vi "Receive Head Tail Location (SubVI).vi"() -> (3 "HT Location":u64[](array[numeric]))   [LabVIEW 2015]
uses:
  <vilib>/rvi/interface/RandomDataEmulation/niFpgaRandomDataHandleErrors.vi
  <vilib>/rvi/DataTransferAndStorage/Container/XNode/niFpgaContainer.xnode
  <vilib>/rvi/interface/RandomDataEmulation/nirviRandomDataFpgaReadWriteTemplate.vi
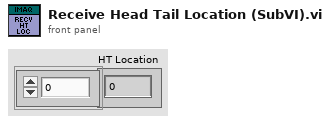
[diagram p1: front panel]
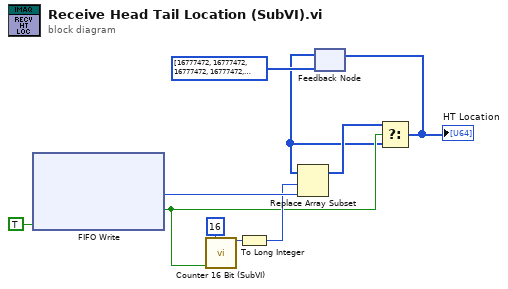
[diagram p0: block diagram]
diagram:
  n1 = xnode ("FIFO Write")("Ready for Output"=TRUE) -> ("Element"=w10:u64, "Output Valid"=w4:bool)  [unwired: 1 in, 1 out]
  n2 = call "Counter 16 Bit (SubVI).vi"("Max. Count"=u16 16, "Enable"=w4) -> ("Count"=w6:u16)  [unwired: 11 in, 2 out]
  n3 = To Long Integer(number=w6) -> (32bit integer=w5:i32)
  n4 = feedback #1(u64[] [16777472, 16777472, 16777472, 16777472, 16777472, 16777472, 16777472, 16777472, 16777472, 16777472, 16777472, 16777472, 16777472, 16777472, 16777472, 16777472] ("HT Location")) -> (w2:u64[])
  n5 = Replace Array Subset(array=w2, new element=w10, index=w5) -> (w9:u64[])
  n6 = Select(t=w9, s=w4, f=w2) -> (s? t:f=w1:u64[])
  "HT Location" <- w1
  n7 = feedback-in #1(w1) -> ()
